vi "ke37xx Configure Scan Arm.vi"(0 "VISA Resource Name":refnum<visa-resource-name>, 7 "Event (0: None)":T1(ring), 11 "error in (no error)":errorcluster) -> (4 "VISA Resource Name Out":refnum<visa-resource-name>, 15 "error out":errorcluster)   [LabVIEW 2009, in "Keithley 3700 Series.lvlib"]
doc: "This VI allows you to set or clear the scan trigger arm event detector."
uses:
  <instrlib>/Keithley 3706/Keithley 3700 Series.lvlib
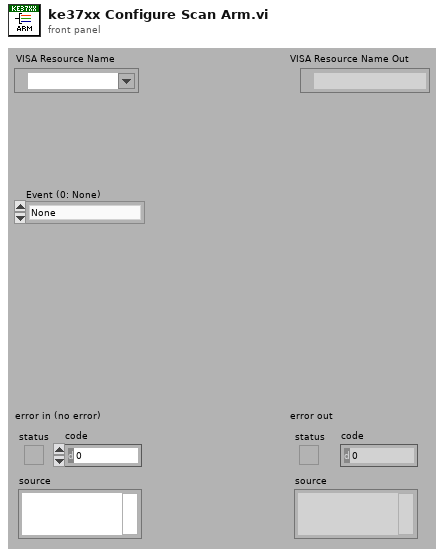
[diagram p1: front panel]
types:
  T1 = enum16{"None", "Alarm 1", "Alarm 2", "Digital I/O Line 1", "Digital I/O Line 2", "Digital I/O Line 3", "Digital I/O Line 4", "Digital I/O Line 5", "Digital I/O Line 6", "Digital I/O Line 7", "Digital I/O Line 8", "Digital I/O Line 9", "Digital I/O Line 10", "Digital I/O Line 11", "Digital I/O Line 12", "Digital I/O Line 13", "Digital I/O Line 14", "TSP Link Line 1", "TSP Link Line 2", "TSP Link Line 3", "Blender 1", "Blender 2", "Timer 1", "Timer 2", "Timer 3", "Timer 4", "LAN Line 1", "LAN Line 2", "LAN Line 3", "LAN Line 4", "LAN Line 5", "LAN Line 6", "LAN Line 7", "LAN Line 8", "DMM Limit 1 High", "DMM Limit 1 Low", "DMM Limit 2 High", "DMM Limit 2 Low", "Display", "Measure Complete", "Sequence Complete", "Scan Ready", "Scan Start", "Scan Complete", "Channel Ready", "Idle", "Software"}
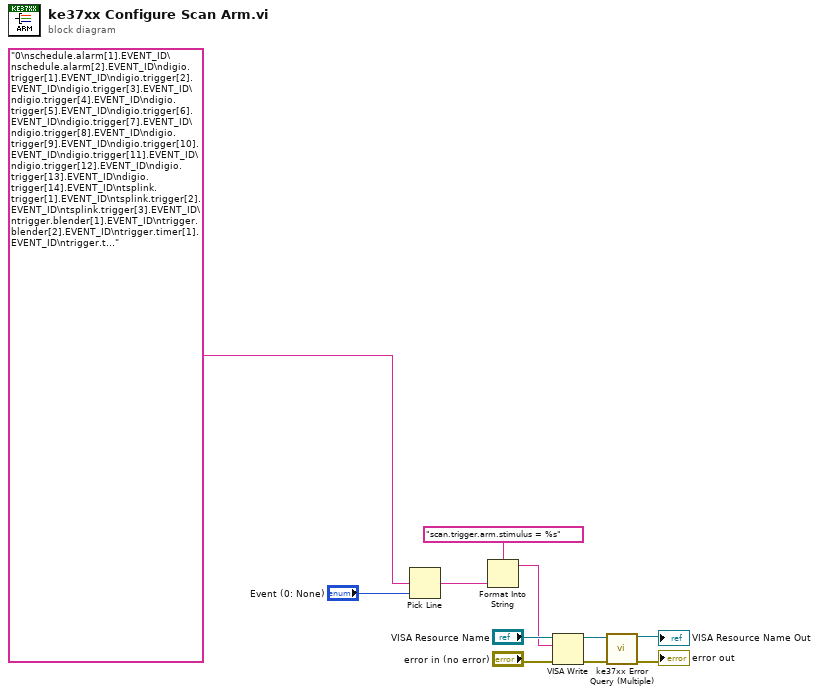
[diagram p0: block diagram]
diagram:
  n1 = Pick Line(multi-line string="0\nschedule.alarm[1].EVENT_ID\nschedule.alarm[2].EVENT_ID\ndigio.trigger[1].EVENT_ID\ndigio.trigger[2].EVENT_ID\ndigio.trigger[3].EVENT_ID\ndigio.trigger[4].EVENT_ID\ndigio.trigger[5].EVENT_ID\ndigio.trigger[6].EVENT_ID\ndigio.trigger[7].EVENT_ID\ndigio.trigger[8].EVENT_ID\ndigio.trigger[9].EVENT_ID\ndigio.trigger[10].EVENT_ID\ndigio.trigger[11].EVENT_ID\ndigio.trigger[12].EVENT_ID\ndigio.trigger[13].EVENT_ID\ndigio.trigger[14].EVENT_ID\ntsplink.trigger[1].EVENT_ID\ntsplink.trigger[2].EVENT_ID\ntsplink.trigger[3].EVENT_ID\ntrigger.blender[1].EVENT_ID\ntrigger.blender[2].EVENT_ID\ntrigger.timer[1].EVENT_ID\ntrigger.timer[2].EVENT_ID\ntrigger.timer[3].EVENT_ID\ntrigger.timer[4].EVENT_ID\nlan.trigger[1].EVENT_ID\nlan.trigger[2].EVENT_ID\nlan.trigger[3].EVENT_ID\nlan.trigger[4].EVENT_ID\nlan.trigger[5].EVENT_ID\nlan.trigger[6].EVENT_ID\nlan.trigger[7].EVENT_ID\nlan.trigger[8].EVENT_ID\ndmm.trigger.EVENT_LIMIT1_HIGH\ndmm.trigger.EVENT_LIMIT1_LOW\ndmm.trigger.EVENT_LIMIT2_HIGH\ndmm.trigger.EVENT_LIMIT2_LOW\ndisplay.trigger.EVENT_ID\nscan.trigger.EVENT_MEASURE_COMP\nscan.trigger.EVENT_SEQUENCE_COMP\nscan.trigger.EVENT_SCAN_READY\nscan.trigger.EVENT_SCAN_START\nscan.trigger.EVENT_SCAN_COMP\nscan.trigger.EVENT_CHANNEL_READY\nscan.trigger.EVENT_IDLE\ntrigger.EVENT_ID", line index="Event (0: None)") -> (output string=w3:string)  [unwired: 1 out]
  n2 = Format Into String(format string="scan.trigger.arm.stimulus = %s", w3) -> (resulting string=w2:string)  [unwired: 2 in, 1 out]
  n3 = VISA Write(VISA resource name="VISA Resource Name", write buffer=w2, error in (no error)="error in (no error)") -> (VISA resource name out=w7:refnum<visa-resource-name>, error out=w6:errorcluster)  [unwired: 1 out]
  n4 = call <instrlib>:"ke37xx Error Query (Multiple).vi"("VISA resource name"=w7, "error in (no error)"=w6) -> ("VISA resource name out"=→"VISA Resource Name Out":refnum<visa-resource-name>, "error out"=→"error out":errorcluster)  [unwired: 12 out]
